vi "Main.vi"() -> ()   [LabVIEW 2017]
uses:
  Steps.ctl
  DAQData.ctl
  <vilib>/Platform/TimedLoop/XDataNode/timing_clust.ctl
  <vilib>/Platform/TimedLoop/XDataNode/nitl_modes.ctl
  <vilib>/Platform/TimedLoop/XDataNode/wakeup.ctl
  <vilib>/Instr/_visa.llb/VISA Configure Serial Port (Instr).vi
  <vilib>/platform/TimedLoop/XDataNode/XDataNode.xnode
  <vilib>/Platform/TimedLoop/XDataNode/XDNodeRunTimeDep.lvlib
panel:
  in  "Tab Control":enum32{"Wait Tab", "Manual Tab", "Running Tab"}(tab)
  in  "Stop":bool
  in  "Manual":bool
  in  "Start":bool
  in  "Arduino COM":refnum<visa-resource-name>="COM8"
  in  "Postition to Be Set":i32[](array[numeric])
  in  "Send Position":bool
  in  "Stop Manual":bool
  out "Sending Position":bool=TRUE
  out "Expected Checksum":i32
  out "Received Checksum":i32
  out "XY Graph":cluster{"Y":dbl[], "Y":dbl[]}[](graph)
  in  "Reset":bool
  in  "Save Button":bool
  in  "Pause":bool
  in  "Run":bool
  in  "Stop Testing":bool
  out "Homing Output":enum16{"Error", "NACK", "ACK", "First Send"}(ring)
  out "Current Position":string[][](array[string])
  in  ".txt Title":string
  out "concatenated string":string
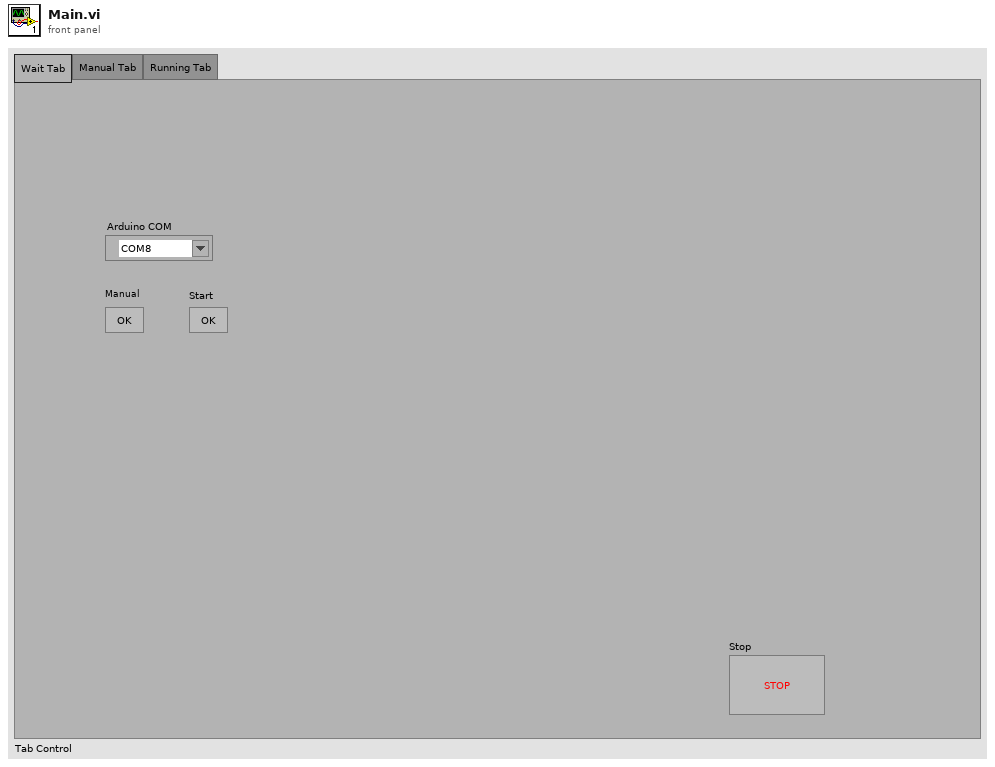
[diagram p1: front panel]
types:
  T1 = typedef "DAQData.ctl" = cluster{"DAQ Data":dbl, "Time Stamp":timestamp, "Y Scale":dbl, "X Scale":dbl, "Position":i32[], "Frequency":dbl}
  T2 = typedef "Steps.ctl" = cluster{"Current Position":i32[], "Steps Increment":i32[], "Steps to Add ":i32[], "Final Position":i32[]}
  T3 = enum16{"Manual", "Testing", "Homing", "Stop", "End Testing", "Wait"}
  T4 = enum8{"Enabled", "Disabled", "Disabled and Grayed Out"}
  T5 = typedef "XDNodeRunTimeDep.lvlib/timing_clust.ctl" = cluster{"Expected End [f-1]":u64, "Actual End [f-1]":u64, "Finished Late? [f-1]":bool, "Expected End [i-1]":u64, "Actual End [i-1]":u64, "Finished Late? [i-1]":bool, "Expected Start [i]":u64, "Actual Start [i]":u64, "Expected Start [f]":u64, "Actual Start [f]":u64, "Source Name":string, "Structure Name":string, "Period":i64, "Deadline":i64, "Offset":i64, "Start":i64, "Priority":i32, "Timeout":i32, "Mode":T6, "Wakeup Reason":T7, "Error":errorcluster, "Source Type":string, "Secondary Source Type":string, "Global End Time":u64, "Global Start Time":u64, "Frame Duration":u64, "Iteration Duration":u64, "Assigned CPU":i32, "I/O Scan Engine Mode":u32}
  T6 = typedef "XDNodeRunTimeDep.lvlib/nitl_modes.ctl" = enum32{"No Change", "Process missed periods, maintain original phase", "Discard missed periods, maintain original phase", "Process missed periods, ignore original phase", "Discard missed periods, ignore original phase"}
  T7 = typedef "XDNodeRunTimeDep.lvlib/wakeup.ctl" = enum32{"Normal", "Aborted", "Asynchronous wakeup", "Timing source error", "Timed loop error", "Timeout"}
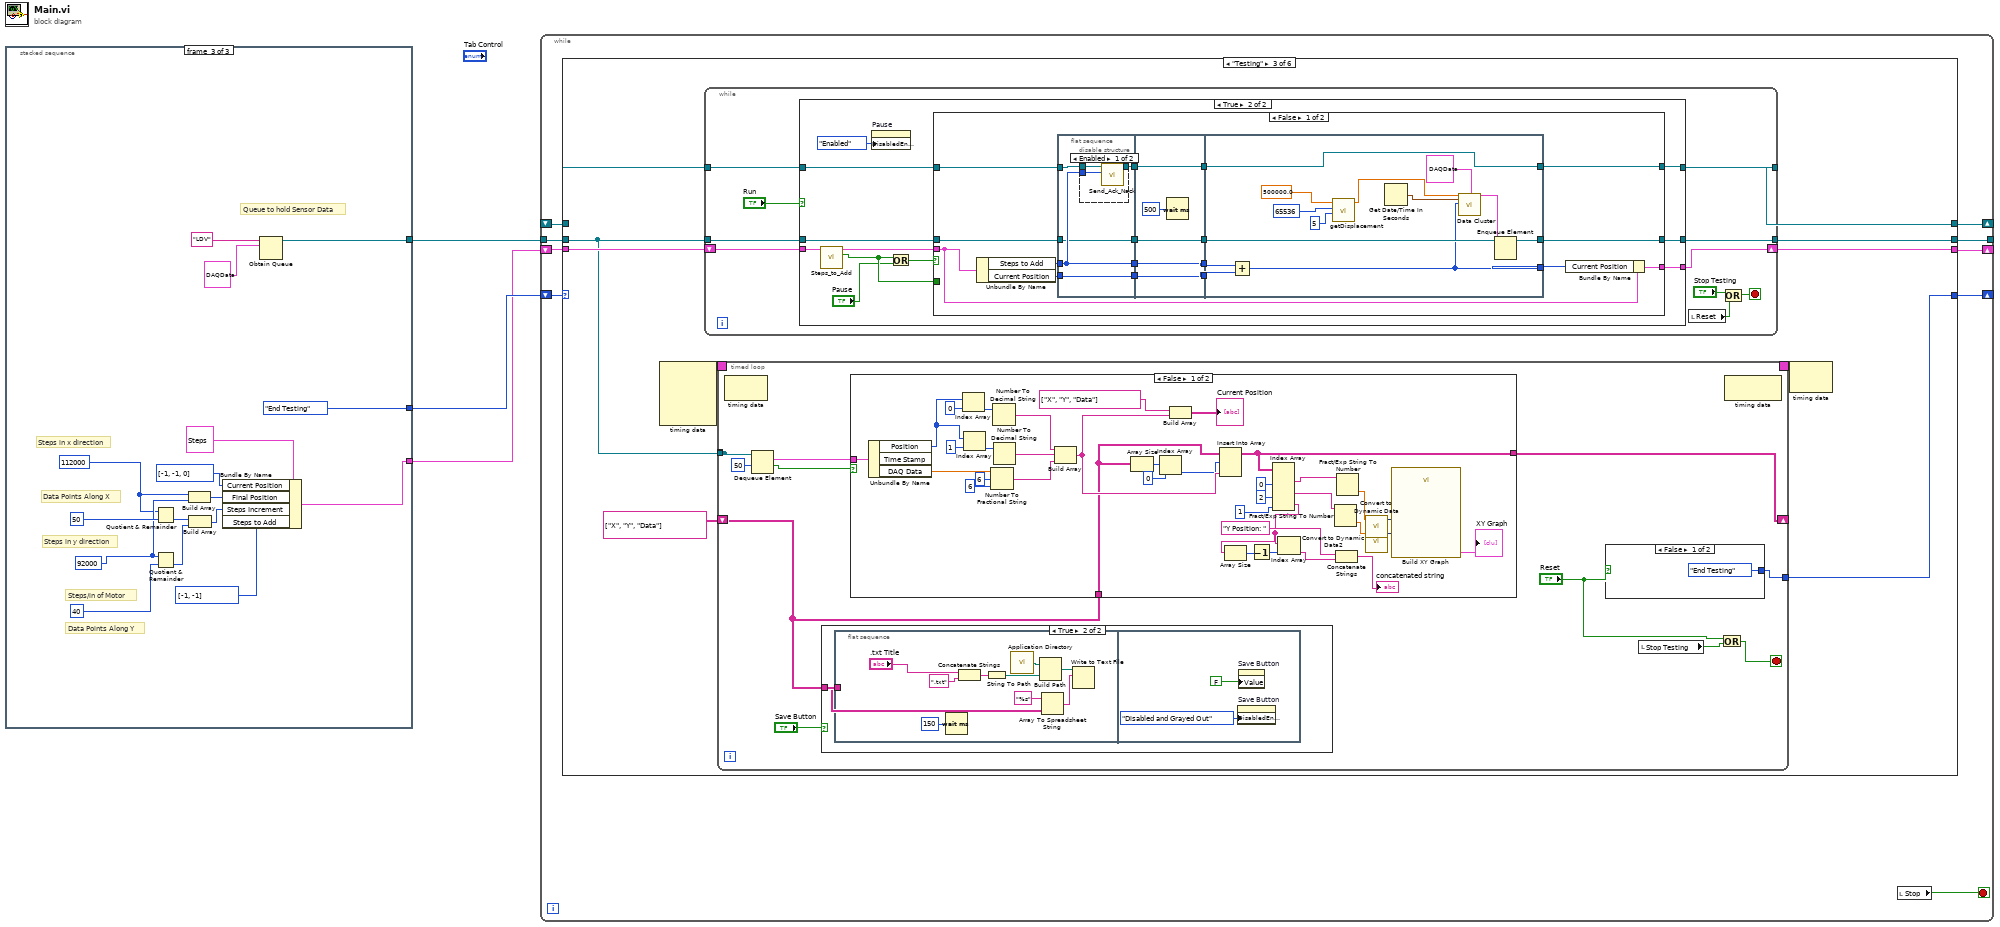
[diagram p0: block diagram]
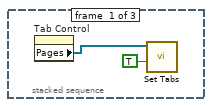
[diagram p2: hidden frame]
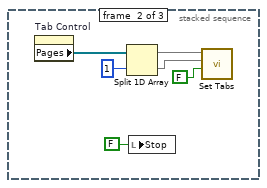
[diagram p3: hidden frame]
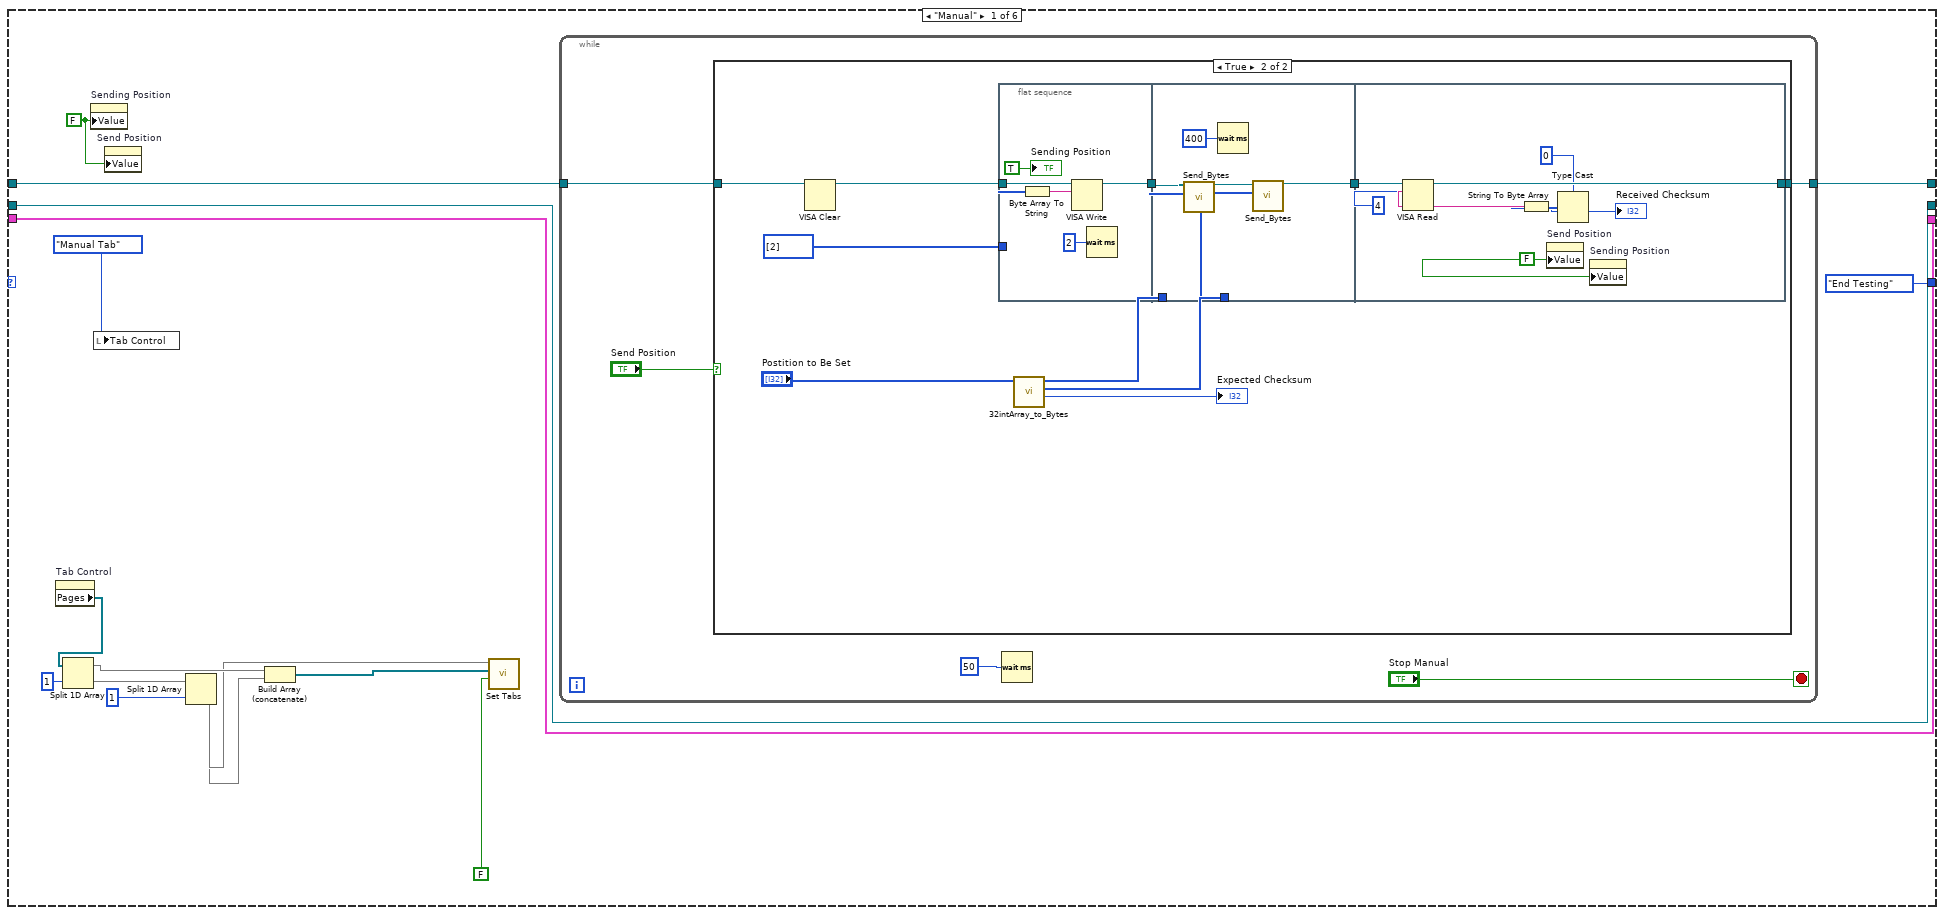
[diagram p4: hidden frame]
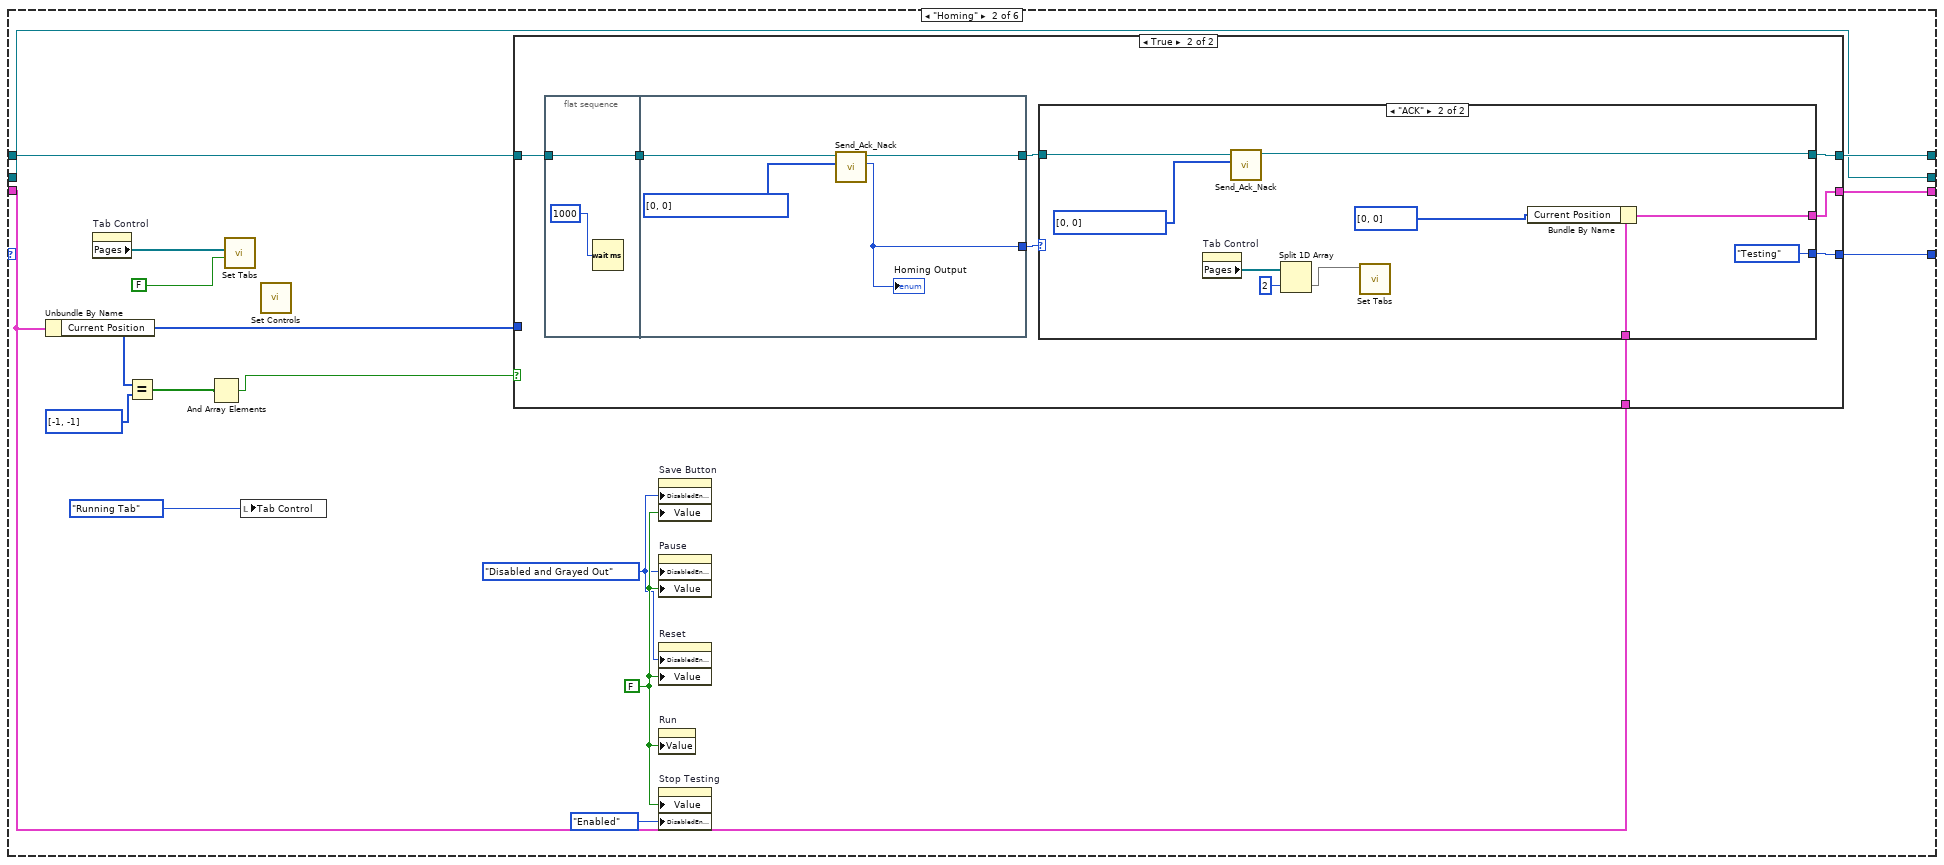
[diagram p6: hidden frame]
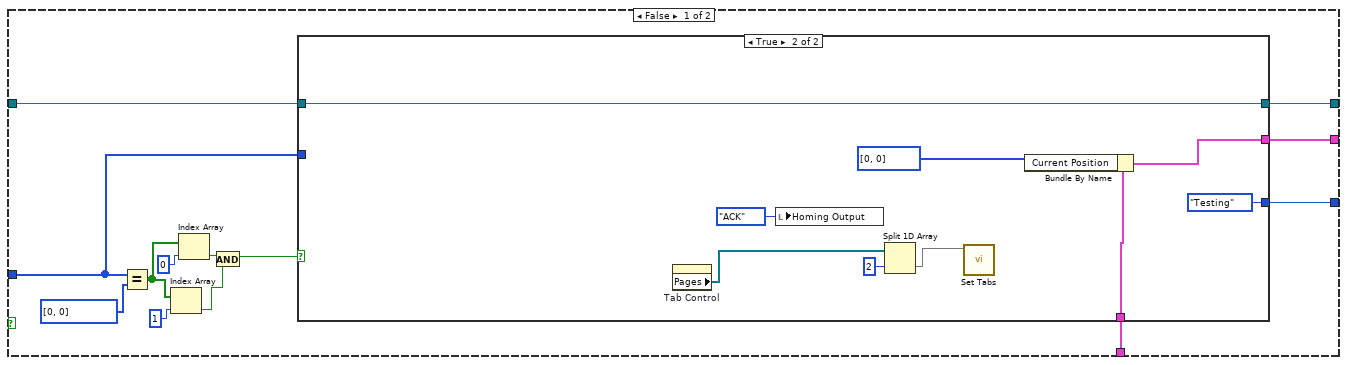
[diagram p7: hidden frame]
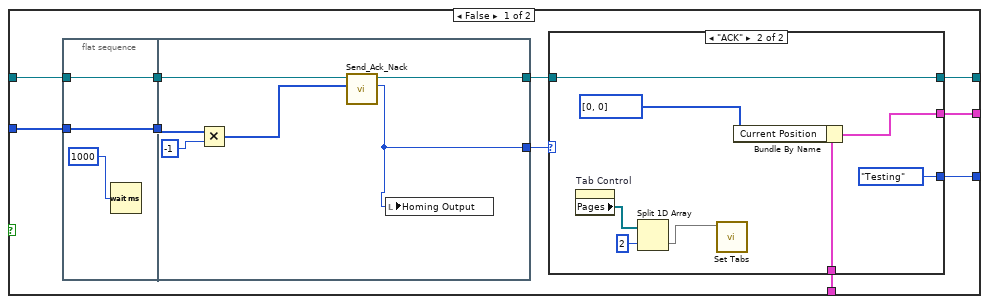
[diagram p8: hidden frame]
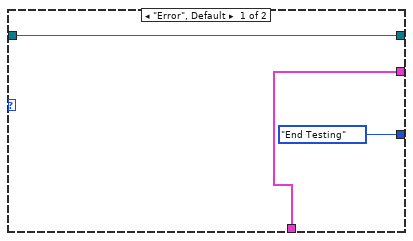
[diagram p9: hidden frame]
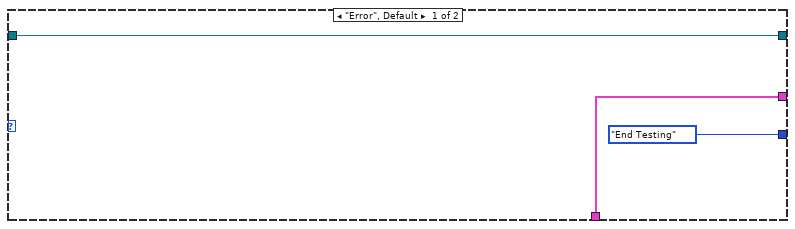
[diagram p10: hidden frame]
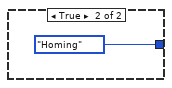
[diagram p13: hidden frame]
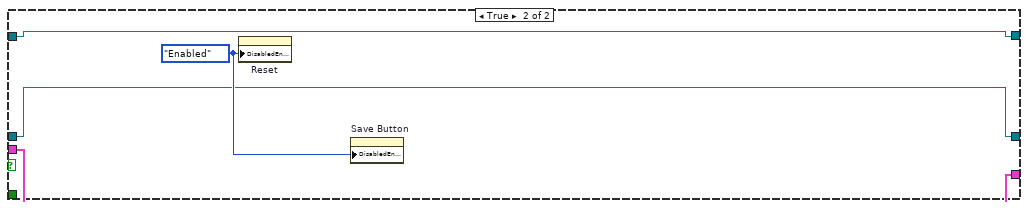
[diagram p16: hidden frame]
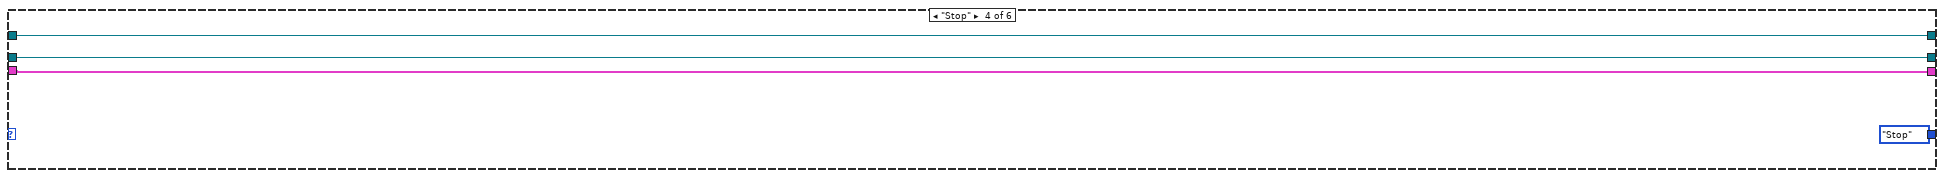
[diagram p17: hidden frame]
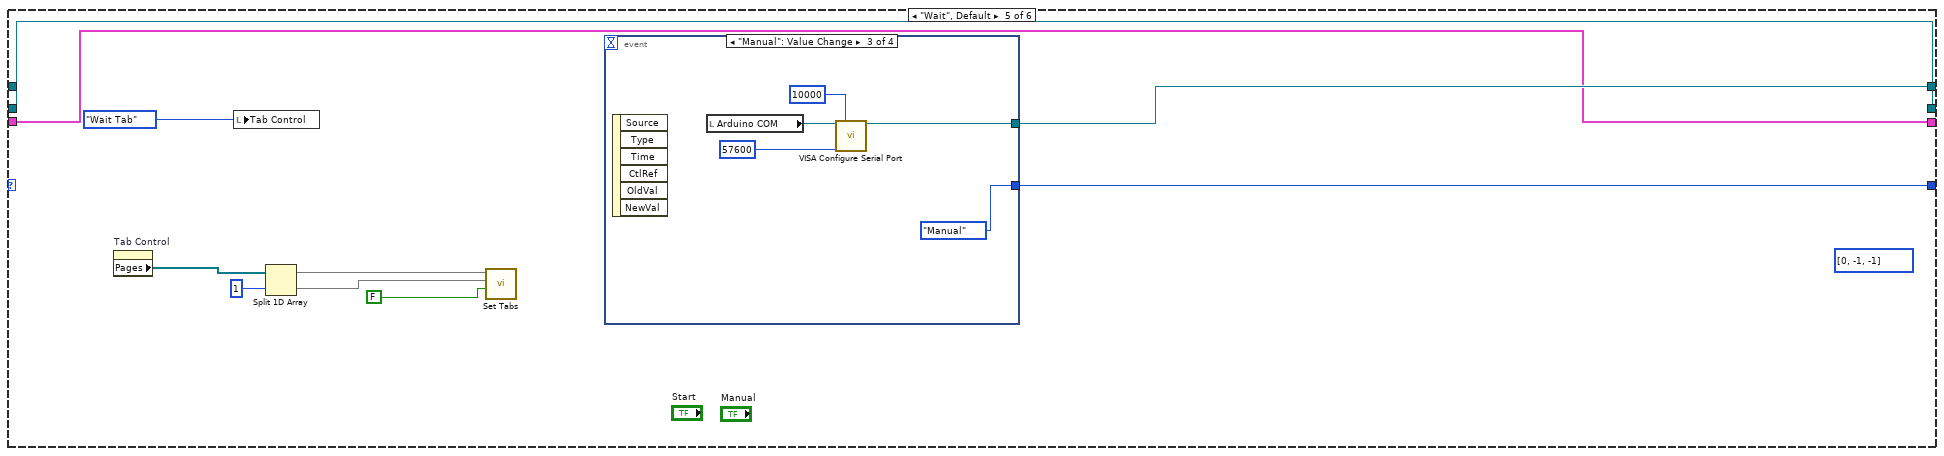
[diagram p18: hidden frame]
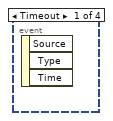
[diagram p19: hidden frame]
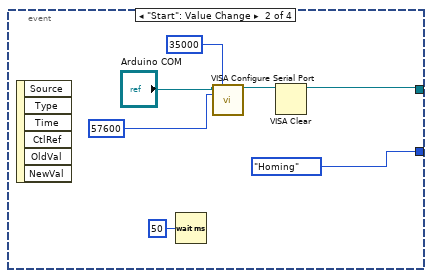
[diagram p20: hidden frame]
diagram:
  n1 = stacked-sequence {
    tunnel: [_ _ T3."End Testing"] -> w3
    tunnel: [_ _ w12] -> w2
    tunnel: [_ _ w18] -> w1
    frame #0 {
      n2 = property on="Tab Control" class="TabCtl (strict)"() -> ("Pages"=w5:refnum<vi>[])  [unwired: 2 in, 2 out]
      n3 = call "Set Tabs.vi"("Enable/Disable Controls?"=TRUE, "Pages To Be Enabled"=w5) -> ()  [unwired: 10 in]
    }
    frame #1 {
      n4 = property on="Tab Control" class="TabCtl (strict)"() -> ("Pages"=w7:refnum<vi>[])  [unwired: 2 in, 2 out]
      n5 = Split 1D Array(array=w7, index=1) -> (first subarray=w9:refnum<vi>[], second subarray=w8:refnum<vi>[])
      n6 = local write "Stop"(FALSE ("Stop")) -> ()
      n7 = call "Set Tabs.vi"("Enable/Disable Controls?"=FALSE, "Pages To Be Disabled"=w8, "Pages To Be Enabled"=w9) -> ()  [unwired: 9 in]
    }
    frame #2 {
      w16 = 92000
      w15 = 112000
      # "Steps in y direction"
      # "Data Points Along Y"
      # "Steps/in of Motor"
      # "Data Points Along X"
      # "Steps in x direction"
      # "Queue to hold Sensor Data"
      n8 = Quotient & Remainder(x=w15, y=50) -> (floor(x/y)=w22:i32)  [unwired: 1 out]
      n9 = Quotient & Remainder(x=w16, y=40) -> (floor(x/y)=w20:i32)  [unwired: 1 out]
      n10 = Build Array(w15, w16) -> (w19:i32[])
      n11 = Build Array(w22, w20) -> (w14:i32[])
      n12 = Bundle By Name(cluster=T2 {"Current Position"=[-1, -1, 0], "Steps Increment"=[-1, -1, 0], "Steps to Add "=[-1, -1, 0], "Final Position"=[-1, -1, 0]}, "Current Position"=i32[] [-1, -1, 0], "Final Position"=w19, "Steps Increment"=w14, "Steps to Add"=i32[] [-1, -1]) -> (w12:T2)
      n13 = Obtain Queue(name (unnamed)="LDV", element data type=T1 {"DAQ Data"=0.0, "Time Stamp"=timestamp(0 s since 1904-01-01), "Y Scale"=0.0, "X Scale"=0.0, "Position"=[], "Frequency"=0.0}) -> (queue out=w18:refnum<queue>)  [unwired: 3 in, 2 out]
    }
  }
  n14 = while {
    shift-right: [w32] -> _
    shift-left: w3 -> [w35]
    shift-right: [w34] -> _
    shift-left: _ -> [w33]
    shift-right: [w28] -> _
    shift-left: w2 -> [w31]
    tunnel: w1 -> [w30]
    tunnel: [w29] -> _
    stop <- w36 stop-if-true
    n15 = case shown="\"Testing\"" w35 {
      tunnel: [w43 w99 w192 w336 w346 _] -> w34
      tunnel: w33 -> [w52 w102 w193 w336 _ w365]
      tunnel: [T3."End Testing" w100 w185 T3."Stop" w339 T3."Wait"] -> w32
      tunnel: w31 -> [w38 w93 w191 w334 w337 w362]
      tunnel: w30 -> [w37 w91 w188 w333 w338 w361]
      tunnel: [w37 w91 w187 w333 w338 w361] -> w29
      tunnel: [w38 w92 w186 w334 w337 w362] -> w28
      frame "Manual" {
        w45 = FALSE ("Sending Position")
        n16 = property on="Tab Control" class="TabCtl (strict)"() -> ("Pages"=w50:refnum<vi>[])  [unwired: 2 in, 2 out]
        n17 = Split 1D Array(array=w50, index=1) -> (first subarray=w48:refnum<vi>[], second subarray=w47:refnum<vi>[])
        n18 = property on="Sending Position" class="Bool (strict)"("Value"=w45) -> ()  [unwired: 2 in, 2 out]
        n19 = local write "Tab Control"(enum32{"Wait Tab", "Manual Tab"}."Manual Tab" ("Tab Control")) -> ()
        n20 = property on="Send Position" class="Bool (strict)"("Value"=w45) -> ()  [unwired: 2 in, 2 out]
        n21 = Split 1D Array(array=w47, index=1) -> (first subarray=w41:refnum<vi>[], second subarray=w39:refnum<vi>[])
        n22 = Build Array (concatenate)(w48, w39) -> (w40:refnum<vi>[])
        n23 = call "Set Tabs.vi"("Enable/Disable Controls?"=FALSE, "Pages To Be Disabled"=w40, "Pages To Be Enabled"=w41) -> ()  [unwired: 9 in]
        n24 = while {
          tunnel: w52 -> [w57]
          tunnel: [w53] -> w43
          stop <- "Stop Manual" stop-if-true
          n25 = case shown="True" "Send Position" {
            tunnel: w57 -> [w58 w68]
            tunnel: [w58 w67] -> w53
            frame False {
            }
            frame True {
              n26 = VISA Clear(VISA resource name=w68) -> (VISA resource name out=w65:refnum<visa-resource-name>)  [unwired: 1 in, 1 out]
              n27 = flat-sequence {
                tunnel: [w74] -> w66
                tunnel: w65 -> [w73]
                tunnel: u8[] [2] -> [w70]
                tunnel: w66 -> [w75]
                tunnel: w63 -> [w77]
                tunnel: [w78] -> w59
                tunnel: w64 -> [w80]
                tunnel: [w87] -> w67
                tunnel: w59 -> [w88]
                frame #0 {
                  n28 = Byte Array To String(unsigned byte array=w70) -> (string=w69:string)
                  n29 = VISA Write(VISA resource name=w73, write buffer=w69) -> (VISA resource name out=w74:refnum<visa-resource-name>)  [unwired: 1 in, 2 out]
                  n30 = Wait (ms)(milliseconds to wait=u32 2) -> ()  [unwired: 1 out]
                  "Sending Position" <- TRUE ("Sending Position")
                }
                frame #1 {
                  n31 = call "Send_Bytes.vi"("Array1"=w80, "VISA resource name"=w75) -> ("VISA resource"=w79:refnum<visa-resource-name>)  [unwired: 9 in]
                  n32 = Wait (ms)(milliseconds to wait=u32 400) -> ()  [unwired: 1 out]
                  n33 = call "Send_Bytes.vi"("Array1"=w77, "VISA resource name"=w79) -> ("VISA resource"=w78:refnum<visa-resource-name>)  [unwired: 9 in]
                }
                frame #2 {
                  w86 = FALSE ("Send Position")
                  n34 = VISA Read(VISA resource name=w88, byte count=u32 4) -> (VISA resource name out=w87:refnum<visa-resource-name>, read buffer=w85:string)  [unwired: 1 in, 2 out]
                  n35 = String To Byte Array(string=w85) -> (unsigned byte array=w84:u8[])
                  n36 = property on="Send Position" class="Bool (strict)"("Value"=w86) -> ()  [unwired: 2 in, 2 out]
                  n37 = Type Cast(type=0, x=w84) -> (*(type *) &x=→"Received Checksum":i32)
                  n38 = property on="Sending Position" class="Bool (strict)"("Value"=w86) -> ()  [unwired: 2 in, 2 out]
                }
              }
              n39 = call "32intArray_to_Bytes.vi"("Postition to Be Set"="Postition to Be Set") -> ("result"=→"Expected Checksum":i32, "Array2"=w63:u8[], "Array1"=w64:u8[])  [unwired: 8 in]
            }
          }
          n40 = Wait (ms)(milliseconds to wait=u32 50) -> ()  [unwired: 1 out]
        }
      }
      frame "Homing" {
        w94 = T4."Disabled and Grayed Out" ("Disabled")
        w95 = FALSE ("Run")
        n41 = Unbundle By Name(w93) -> ("Current Position"=w96:i32[])
        n42 = property on="Tab Control" class="TabCtl (strict)"() -> ("Pages"=w101:refnum<vi>[])  [unwired: 2 in, 2 out]
        n43 = Equal?(x=w96, y=i32[] [-1, -1]) -> (x = y?=w90:bool[])
        n44 = And Array Elements(Boolean array=w90) -> (logical AND=w89:bool)
        n45 = call "Set Tabs.vi"("Enable/Disable Controls?"=FALSE, "Pages To Be Disabled"=w101) -> ()  [unwired: 10 in]
        n46 = local write "Tab Control"(enum32{"Wait Tab", "Manual Tab", "Running Tab"}."Running Tab" ("Tab Control")) -> ()
        n47 = call "Set Controls.vi"() -> ()  [unwired: 3 in]
        n48 = case shown="True" w89 {
          tunnel: w102 -> [w110 w163]
          tunnel: [w107 w162] -> w100
          tunnel: [w109 w159] -> w99
          tunnel: w96 -> [w108 _]
          tunnel: w93 -> [w106 w158]
          tunnel: [w105 w157] -> w92
          frame False {
            n49 = Equal?(x=w108, y=i32[] [0, 0]) -> (x = y?=w113:bool[])
            n50 = Index Array(array=w113, index=1) -> (element=w115:bool)
            n51 = Index Array(array=w113, index=0) -> (element=w112:bool)
            n52 = And(x=w112, y=w115) -> (x .and. y?=w111:bool)
            n53 = case shown="True" w111 {
              tunnel: w110 -> [w127 w156]
              tunnel: [w121 w156] -> w109
              tunnel: w108 -> [w125 _]
              tunnel: [w120 T3."Testing"] -> w107
              tunnel: w106 -> [w119 w153]
              tunnel: [w118 w152] -> w105
              frame False {
                n54 = flat-sequence {
                  tunnel: w127 -> [w140]
                  tunnel: [w140] -> w126
                  tunnel: w125 -> [w139]
                  tunnel: [w139] -> w124
                  tunnel: [w142] -> w123
                  tunnel: [w147] -> w122
                  tunnel: w126 -> [w146]
                  tunnel: w124 -> [w145]
                  frame #0 {
                    n55 = Wait (ms)(milliseconds to wait=u32 1000) -> ()  [unwired: 1 out]
                  }
                  frame #1 {
                    n56 = Multiply(x=w145, y=-1) -> (x*y=w143:i32[])
                    n57 = call "Send_Ack_Nack.vi"("Postition to Be Set in"=w143, "VISA resource name"=w146) -> ("Output"=w142:enum16{"Error", "NACK", "ACK", "First Send"}, "VISA Out"=w147:refnum<visa-resource-name>)  [unwired: 6 in]
                    n58 = local write "Homing Output"(w142) -> ()
                  }
                }
                n59 = case shown="\"ACK\"" w123 {
                  tunnel: w122 -> [w130 w137]
                  tunnel: [w130 w137] -> w121
                  tunnel: [T3."End Testing" T3."Testing"] -> w120
                  tunnel: w119 -> [w128 w135]
                  tunnel: [w128 w134] -> w118
                  frame "Error", Default {
                  }
                  frame "ACK" {
                    n60 = property on="Tab Control" class="TabCtl (strict)"() -> ("Pages"=w131:refnum<vi>[])  [unwired: 2 in, 2 out]
                    n61 = Split 1D Array(array=w131, index=2) -> (second subarray=w132:refnum<vi>[])  [unwired: 1 out]
                    n62 = call "Set Tabs.vi"("Pages To Be Enabled"=w132) -> ()  [unwired: 11 in]
                    n63 = Bundle By Name(cluster=w135, "Current Position"=i32[] [0, 0]) -> (w134:T2)
                  }
                }
              }
              frame True {
                n64 = property on="Tab Control" class="TabCtl (strict)"() -> ("Pages"=w148:refnum<vi>[])  [unwired: 2 in, 2 out]
                n65 = local write "Homing Output"(enum16{"Error", "NACK", "ACK", "First Send"}."ACK" ("Homing Output")) -> ()
                n66 = Split 1D Array(array=w148, index=2) -> (second subarray=w149:refnum<vi>[])  [unwired: 1 out]
                n67 = call "Set Tabs.vi"("Pages To Be Enabled"=w149) -> ()  [unwired: 11 in]
                n68 = Bundle By Name(cluster=w153, "Current Position"=i32[] [0, 0]) -> (w152:T2)
              }
            }
          }
          frame True {
            n69 = flat-sequence {
              tunnel: w163 -> [w166]
              tunnel: [w166] -> w164
              tunnel: [w168] -> w161
              tunnel: [w167] -> w160
              tunnel: w164 -> [w170]
              frame #0 {
                n70 = Wait (ms)(milliseconds to wait=u32 1000) -> ()  [unwired: 1 out]
              }
              frame #1 {
                n71 = call "Send_Ack_Nack.vi"("Postition to Be Set in"=i32[] [0, 0], "VISA resource name"=w170) -> ("Output"=w168:enum16{"Error", "NACK", "ACK", "First Send"}, "VISA Out"=w167:refnum<visa-resource-name>)  [unwired: 6 in]
                "Homing Output" <- w168
              }
            }
            n72 = case shown="\"ACK\"" w161 {
              tunnel: [T3."End Testing" T3."Testing"] -> w162
              tunnel: [w172 w181] -> w159
              tunnel: w160 -> [w172 w182]
              tunnel: w158 -> [w171 w176]
              tunnel: [w171 w174] -> w157
              frame "Error", Default {
              }
              frame "ACK" {
                n73 = property on="Tab Control" class="TabCtl (strict)"() -> ("Pages"=w179:refnum<vi>[])  [unwired: 2 in, 2 out]
                n74 = call "Send_Ack_Nack.vi"("Postition to Be Set in"=i32[] [0, 0], "VISA resource name"=w182) -> ("VISA Out"=w181:refnum<visa-resource-name>)  [unwired: 6 in, 1 out]
                n75 = Split 1D Array(array=w179, index=2) -> (second subarray=w177:refnum<vi>[])  [unwired: 1 out]
                n76 = call "Set Tabs.vi"("Pages To Be Enabled"=w177) -> ()  [unwired: 11 in]
                n77 = Bundle By Name(cluster=w176, "Current Position"=i32[] [0, 0]) -> (w174:T2)
              }
            }
          }
        }
        n78 = property on="Save Button" class="Bool (strict)"("DisabledEnum"=w94, "Value"=w95) -> ()  [unwired: 2 in, 2 out]
        n79 = property on="Pause" class="Bool (strict)"("DisabledEnum"=w94, "Value"=w95) -> ()  [unwired: 2 in, 2 out]
        n80 = property on="Reset" class="Bool (strict)"("DisabledEnum"=w94, "Value"=w95) -> ()  [unwired: 2 in, 2 out]
        n81 = property on="Run" class="Bool (strict)"("Value"=w95) -> ()  [unwired: 2 in, 2 out]
        n82 = property on="Stop Testing" class="Bool (strict)"("Value"=w95, "DisabledEnum"=T4."Enabled" ("Disabled")) -> ()  [unwired: 2 in, 2 out]
      }
      frame "Testing" {
        n83 = node-c288() -> (w190:T5)  [unwired: 4 in]
        n84 = while {
          tunnel: w193 -> [w270]
          tunnel: [w268] -> w192
          tunnel: w188 -> [w266]
          tunnel: [w265] -> w187
          shift-right: [w264] -> w186
          shift-left: w191 -> [w267]
          stop <- w262 stop-if-true
          n85 = case shown="True" "Run" {
            tunnel: w270 -> [w273 w280]
            tunnel: w267 -> [w271 w284]
            tunnel: [w273 w279] -> w268
            tunnel: w266 -> [w272 w278]
            tunnel: [w272 w277] -> w265
            tunnel: [w271 w276] -> w264
            frame False {
            }
            frame True {
              n86 = call "Steps_to_Add.vi"("Cluster"=w284) -> ("logical AND"=w275:bool, "output cluster"=w281:T2)  [unwired: 9 in]
              n87 = property on="Pause" class="Bool (strict)"("DisabledEnum"=T4."Enabled" ("Disabled")) -> ()  [unwired: 2 in, 2 out]
              n88 = Or(x=w275, y="Pause") -> (x .or. y?=w282:bool)
              n89 = case shown="False" w282 {
                tunnel: w281 -> [w295 w330]
                tunnel: w280 -> [w299 w329]
                tunnel: [w298 w329] -> w279
                tunnel: w278 -> [w297 w331]
                tunnel: [w296 w331] -> w277
                tunnel: [w293 w330] -> w276
                tunnel: w275 -> [_ _]
                frame False {
                  n90 = Unbundle By Name(w295) -> ("Steps to Add"=w300:i32[], "Current Position"=w301:i32[])
                  n91 = flat-sequence {
                    tunnel: w301 -> [w304]
                    tunnel: w300 -> [w305]
                    tunnel: w299 -> [w306]
                    tunnel: [w305] -> w292
                    tunnel: [w304] -> w290
                    tunnel: [w303] -> w288
                    tunnel: w297 -> [w302]
                    tunnel: [w302] -> w286
                    tunnel: w292 -> [w315]
                    tunnel: [w315] -> w291
                    tunnel: w290 -> [w314]
                    tunnel: [w314] -> w289
                    tunnel: w288 -> [w313]
                    tunnel: [w313] -> w287
                    tunnel: w286 -> [w312]
                    tunnel: [w312] -> w285
                    tunnel: w291 -> [w328]
                    tunnel: w289 -> [w327]
                    tunnel: [w326] -> w298
                    tunnel: w287 -> [w326]
                    tunnel: w285 -> [w325]
                    tunnel: [w322] -> w294
                    tunnel: [w320] -> w296
                    frame #0 {
                      n92 = disable-structure shown="Enabled" {
                        disable-tunnel: w306 -> [w309 w310]
                        disable-tunnel: w305 -> [w308 _]
                        disable-tunnel: [w307 w310] -> w303
                        frame Enabled {
                          n93 = call "Send_Ack_Nack.vi"("Postition to Be Set in"=w308, "VISA resource name"=w309) -> ("VISA Out"=w307:refnum<visa-resource-name>)  [unwired: 6 in, 1 out]
                        }
                        frame Disabled {
                        }
                      }
                    }
                    frame #1 {
                      n94 = Wait (ms)(milliseconds to wait=u32 500) -> ()  [unwired: 1 out]
                    }
                    frame #2 {
                      n95 = Add(x=w328, y=w327) -> (x+y=w322:i32[])
                      n96 = call "getDisplacement.vi"("Samples to Average"=5, "Samples"=65536, "Sampling Frequency"=500000.0) -> ("max value"=w316:dbl)  [unwired: 8 in]
                      n97 = Get Date/Time In Seconds() -> (seconds since 1Jan1904=w324:timestamp)
                      n98 = call "Data Cluster.vi"("DAQ Data"=w316, "seconds since 1Jan1904"=w324, "Array"=w322, "Cluster in"=T1 {"DAQ Data"=0.0, "Time Stamp"=timestamp(0 s since 1904-01-01), "Y Scale"=0.0, "X Scale"=0.0, "Position"=[], "Frequency"=0.0}) -> ("Cluster out"=w321:T1)  [unwired: 15 in]
                      n99 = Enqueue Element(queue=w325, element=w321) -> (queue out=w320:refnum<queue>)  [unwired: 2 in, 2 out]
                    }
                  }
                  n100 = Bundle By Name(cluster=w295, "Current Position"=w294) -> (w293:T2)
                }
                frame True {
                  w332 = T4."Enabled" ("Disabled")
                  n101 = property on="Reset" class="Bool (strict)"("DisabledEnum"=w332) -> ()  [unwired: 2 in, 2 out]
                  n102 = property on="Save Button" class="Bool (strict)"("DisabledEnum"=w332) -> ()  [unwired: 2 in, 2 out]
                }
              }
            }
          }
          n103 = local read "Reset"() -> (w261:bool)
          n104 = Compound Arithmetic op=OR("Stop Testing", w261) -> (w262:bool)
        }
        n105 = timed-loop {
          timing: w190 -> [_]
          timing-out: [_] -> w189
          tunnel: [w199] -> _
          tunnel: w188 -> [w199]
          tunnel: [w201] -> w185
          shift-right: [w195] -> _
          shift-left: string[][] [["X", "Y", "Data"]] -> [w194]
          stop <- w204 stop-if-true
          n106 = node-c288() -> ()  [unwired: 1 in, 1 out]
          n107 = Dequeue Element(queue=w199, timeout in ms (-1)=50) -> (element=w198:T1, timed out?=w197:bool)  [unwired: 1 in, 2 out]
          n108 = case shown="True" "Save Button" {
            tunnel: w194 -> [_ w242]
            frame False {
            }
            frame True {
              n109 = flat-sequence {
                tunnel: w242 -> [w245]
                frame #0 {
                  n110 = Wait (ms)(milliseconds to wait=u32 150) -> ()  [unwired: 1 out]
                  n111 = Concatenate Strings(".txt Title", ".txt" ("string")) -> (w250:string)
                  n112 = String To Path(string=w250) -> (path=w249:path)
                  n113 = call <vilib>:"Application Directory.vi"() -> ("Application Directory"=w251:path)
                  n114 = Build Path(base path=w251, name or relative path=w249) -> (appended path=w246:path)
                  n115 = Array To Spreadsheet String(array=w245, 3:"%s" ("format string")) -> (spreadsheet string=w247:string)  [unwired: 1 in]
                  n116 = Write to Text File(file (use dialog)=w246, text=w247) -> ()  [unwired: 2 in, 3 out]
                }
                frame #1 {
                  n117 = property on="Save Button" class="Bool (strict)"("DisabledEnum"=T4."Disabled and Grayed Out" ("Disabled")) -> ()  [unwired: 2 in, 2 out]
                  n118 = property on="Save Button" class="Bool (strict)"("Value"=FALSE ("Save Button")) -> ()  [unwired: 2 in, 2 out]
                }
              }
            }
          }
          n119 = case shown="False" w197 {
            tunnel: w198 -> [w240 _]
            tunnel: w194 -> [w229 w241]
            tunnel: [w220 w241] -> w195
            frame False {
              n120 = Unbundle By Name(w240) -> ("Position"=w235:i32[], "DAQ Data"=w225:dbl)  [unwired: 1 out]
              n121 = Index Array(array=w235, index=0) -> (element=w237:i32)
              n122 = Index Array(array=w235, index=1) -> (element=w236:i32)
              n123 = Number To Fractional String(number=w225, width (-)=i16 6, precision (6)=i16 6) -> (F-format string=w222:string)  [unwired: 1 in]
              n124 = Number To Decimal String(number=w237) -> (decimal integer string=w234:string)  [unwired: 1 in]
              n125 = Number To Decimal String(number=w236) -> (decimal integer string=w233:string)  [unwired: 1 in]
              n126 = Build Array(w234, w233, w222) -> (w230:string[])
              n127 = Array Size(array=w229) -> (size(s)=w228:i32[])
              n128 = Index Array(array=w228, index=0) -> (element=w226:i32)
              n129 = Build Array(string[] ["X", "Y", "Data"], w230) -> (→"Current Position":string[][])
              n130 = Insert Into Array(array=w229, index (row)=w226, new element=w230) -> (w220:string[][])  [unwired: 1 in]
              n131 = Index Array(array=w220, index (col) #1=0 ("disabled index (col)"), index (col) #2=2 ("index (col)"), index (col) #3=1 ("index (col)")) -> (element #1=w217:string[], element #2=w216:string[], element #3=w208:string[])  [unwired: 3 in]
              n132 = Array Size(array=w208) -> (size(s)=w207:i32)
              n133 = Decrement(x=w207) -> (x-1=w206:i32)
              n134 = Index Array(array=w208, index=w206) -> (element=w209:string)
              n135 = Fract/Exp String To Number(string=w216) -> (number=w213:dbl[])  [unwired: 3 in, 1 out]
              n136 = Concatenate Strings("Y Position: ", w209) -> (→"concatenated string":string)
              n137 = Fract/Exp String To Number(string=w217) -> (number=w215:dbl[])  [unwired: 3 in, 1 out]
              n138 = call "Convert to Dynamic Data"("Array"=w215) -> ("Dynamic Data Type"=w214:dynamicdata)  [unwired: 3 in]
              n139 = call "Convert to Dynamic Data2"("Array"=w213) -> ("Dynamic Data Type"=w205:dynamicdata)  [unwired: 3 in]
              n140 = call "Build XY Graph"("Y Input"=w205, "X Input"=w214) -> ("XY Graph"=→"XY Graph":cluster{"X":dbl[], "Y":dbl[]}[])  [unwired: 8 in, 1 out]
            }
            frame True {
            }
          }
          n141 = case shown="False" "Reset" {
            tunnel: [T3."End Testing" T3."Homing"] -> w201
            frame False {
            }
            frame True {
            }
          }
          n142 = local read "Stop Testing"() -> (w203:bool)
          n143 = Compound Arithmetic op=OR("Reset", w203) -> (w204:bool)
          n144 = node-c288() -> ()  [unwired: 1 in, 1 out]
        }
        n145 = node-c288(w189) -> ()  [unwired: 1 out]
      }
      frame "Stop" {
      }
      frame "Wait", Default {
        (unwired) i32[] [0, -1, -1]
        n146 = property on="Tab Control" class="TabCtl (strict)"() -> ("Pages"=w340:refnum<vi>[])  [unwired: 2 in, 2 out]
        n147 = local write "Tab Control"(enum32{"Wait Tab", "Manual Tab"}."Wait Tab" ("Tab Control")) -> ()
        n148 = Split 1D Array(array=w340, index=1) -> (first subarray=w342:refnum<vi>[], second subarray=w341:refnum<vi>[])
        n149 = call "Set Tabs.vi"("Enable/Disable Controls?"=FALSE, "Pages To Be Disabled"=w341, "Pages To Be Enabled"=w342) -> ()  [unwired: 9 in]
        n150 = event shown="[2] \"Manual\": Value Change" {
          selector: _ -> [_ _ _ _]
          dyn-events: _ -> [_ _ _ _]
          timeout: _ -> [_ _ _ _]
          tunnel: [_ w348 w354 _] -> w346
          tunnel: [_ T3."Homing" T3."Manual" T3."Stop"] -> w339
          event Timeout {
            n151 = event-data() -> ()  [unwired: 1 in, 3 out]
          }
          event "Start": Value Change {
            n152 = event-data() -> ()  [unwired: 1 in, 6 out]
            n153 = Wait (ms)(milliseconds to wait=u32 50) -> ()  [unwired: 1 out]
            n154 = call-poly "VISA Configure Serial Port"("VISA resource name"="Arduino COM", "timeout (10sec)"=u32 35000, "baud rate (9600)"=u32 57600) -> ("VISA resource name out"=w352:refnum<visa-resource-name>)  [unwired: 11 in, 1 out]
            n155 = VISA Clear(VISA resource name=w352) -> (VISA resource name out=w348:refnum<visa-resource-name>)  [unwired: 1 in, 1 out]
          }
          event "Manual": Value Change {
            n156 = event-data() -> ()  [unwired: 1 in, 6 out]
            n157 = local read "Arduino COM"() -> (w358:refnum<visa-resource-name>)
            n158 = call-poly "VISA Configure Serial Port"("VISA resource name"=w358, "timeout (10sec)"=u32 10000, "baud rate (9600)"=u32 57600) -> ("VISA resource name out"=w354:refnum<visa-resource-name>)  [unwired: 11 in, 1 out]
          }
          event "Stop": Value Change {
            n159 = event-data() -> ()  [unwired: 1 in, 6 out]
            n160 = local write "Stop"("Stop") -> ()
          }
        }
      }
      frame "End Testing" {
        w363 = FALSE ("Manual")
        n161 = property on="Manual" class="Bool (strict)"("Value"=w363) -> ()  [unwired: 2 in, 2 out]
        n162 = property on="Start" class="Bool (strict)"("Value"=w363) -> ()  [unwired: 2 in, 2 out]
        n163 = property on="Stop Manual" class="Bool (strict)"("Value"=w363) -> ()  [unwired: 2 in, 2 out]
        n164 = property on="Stop Testing" class="Bool (strict)"("Value"=w363) -> ()  [unwired: 2 in, 2 out]
        n165 = property on="Save Button" class="Bool (strict)"("Value"=w363) -> ()  [unwired: 2 in, 2 out]
        n166 = property on="Pause" class="Bool (strict)"("Value"=w363) -> ()  [unwired: 2 in, 2 out]
        n167 = property on="Reset" class="Bool (strict)"("Value"=w363) -> ()  [unwired: 2 in, 2 out]
        n168 = VISA Close(VISA resource name=w365) -> ()  [unwired: 1 in, 1 out]
      }
    }
    n169 = local read "Stop"() -> (w36:bool)
  }
